vi "register.vi"(0 "HGF_Monitor in":refnum<class "HGF_Monitor.lvclass">, 5 "Variable URL":string, 7 "HGF_NetworkVisitor":refnum<class "HGF_NetworkVisitor.lvclass">, 9 "HGF_TriggeredEvent":refnum<class "HGF_TriggeredEvent.lvclass">, 11 "error in (no error)":errorcluster) -> (4 "HGF_Monitor out":refnum<class "HGF_Monitor.lvclass">, 15 "error out":errorcluster)   [LabVIEW 2012, in "HGF_SV.lvlib" / "HGF_Monitor.lvclass"]
uses:
  HGF_Monitor.lvclass
  HGF_BaseClasses/HGF_NetworkVisitor/HGF_NetworkVisitor.lvclass
  HGF_BaseClasses/HGF_TriggeredEvent/HGF_TriggeredEvent.lvclass
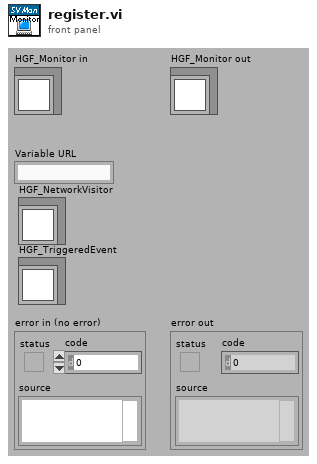
[diagram p1: front panel]
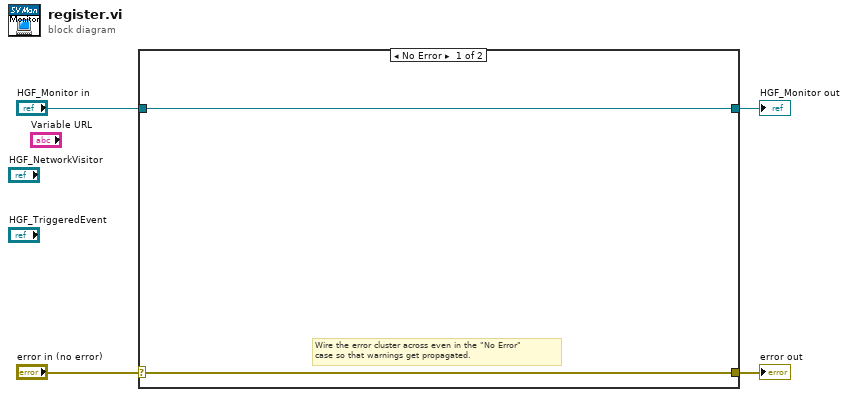
[diagram p0: block diagram]
diagram:
  n1 = case shown="No Error" "error in (no error)" {
    selector: "error in (no error)" -> [w5 w8]
    tunnel: [w5 w8] -> w3
    tunnel: [w6 w7] -> w1
    tunnel: "HGF_Monitor in" -> [w6 w7]
    frame No Error {
      # "Wire the error cluster across even in the \"No Error\"\ncase so that warnings get propagated."
    }
    frame Error {
    }
  }
  "error out" <- w3
  "HGF_Monitor out" <- w1
